vi "oa_TV Set Channel Info (Even Angle Output 1Chan).vi"(0 "seconds/rev":dbl[](array[numeric]) format="%.2f", 1 "torisional vibration unit (RPM)":enum16{"RPM", "deg/s", "rad/s"}(ring), 5 "pulse position":dbl[](array[numeric]), 7 "pulse/revolution (1)":i32=1, 11 "error in (no error)":errorcluster, 12 "r0":dbl, 13 "dr":dbl) -> (4 "even-angle torsional vibration":cluster{"r0":dbl, "dr":dbl, "Y":dbl[]}={"r0"=0.0, "dr"=1.0, "Y"=[]} {"r0" format="%.2p"; "dr" format="%.2p"; "Y" format="%.2f"}, 6 "even-angle channel info":T3={"channel name"="", "description"="", " channel info"={"sensor sensitivity"=1000.0, "engineering units"=1, "dB reference"=1.0, "custom label"="EU", "weighting filter"=0, "pregain"=0.0}} {"channel info"."pregain" format="%.2f"; "channel info"."weighting filter" items=["Linear", "A-weighting", "B-weighting", "C-weighting", "ITU-R 468-4", "Dolby", "CCITT", "C-message", "Wb", "Wc", "Wd", "We", "Wf", "Wh", "Wj", "Wk", "Wm", "AES17 20 kHz lowpass", "AES17 40 kHz lowpass", "AES17 20 kHz highpass", "AES17 40 kHz highpass"]; "channel info"."dB reference" format="%^.1e"; "channel info"."engineering units" items=["custom..."=0, "V"=1, "A"=21, "C"=30, "pC"=31, "s"=32, "-"=29, "Pa"=2, "N"=20, "g"=3, "m/s^2"=4, "m/s"=5, "m"=6, "mm/s"=12, "mm"=13, "micron/s"=14, "micron"=15, "in/s^2"=7, "in/s"=8, "in"=9, "mil/s"=10, "mil"=11, "rad/s^2"=16, "rad/s"=17, "rad"=18, "deg/s^2"=26, "deg/s"=27, "deg"=28, "RPM"=22, "cycle/s^2"=23, "Hz"=24, "cycle"=25, "strain"=19]; "channel info"."sensor sensitivity" format="%#_5f"}, 8 "speed profile":T2 {"speed [RPM]" format="%.2f"; "time [s]" format="%.2f"}, 10 "position info":T1, 14 "unit label":string, 15 "error out":errorcluster)   [LabVIEW 2017, in "SoundVib_Torsional.lvlib"]
uses:
  <vilib>/addons/Sound and Vibration/Order Analysis/Torsional Vibration/SoundVib_Torsional.lvlib
  <vilib>/addons/_NISVFA/_Shared subVIs/Controls/svc_Resampled Channel Info.ctl
  <vilib>/addons/_NISVFA/_Shared subVIs/Controls/svc_Channel Info.ctl
  <vilib>/addons/_NISVFA/_Shared subVIs/Controls/svc_Engineering Units Text Ring.ctl
  <vilib>/addons/_NISVFA/_Shared subVIs/Controls/svc_Weighting Filter Text Ring.ctl
  <vilib>/addons/Sound and Vibration/Order Analysis/Tach Process/SubVIs/speed profile.ctl
  <vilib>/addons/Sound and Vibration/Order Analysis/Misc/OAT Position Info.ctl
  <vilib>/addons/Sound and Vibration/Order Analysis/Tach Process/SoundVib_TachProcess.lvlib
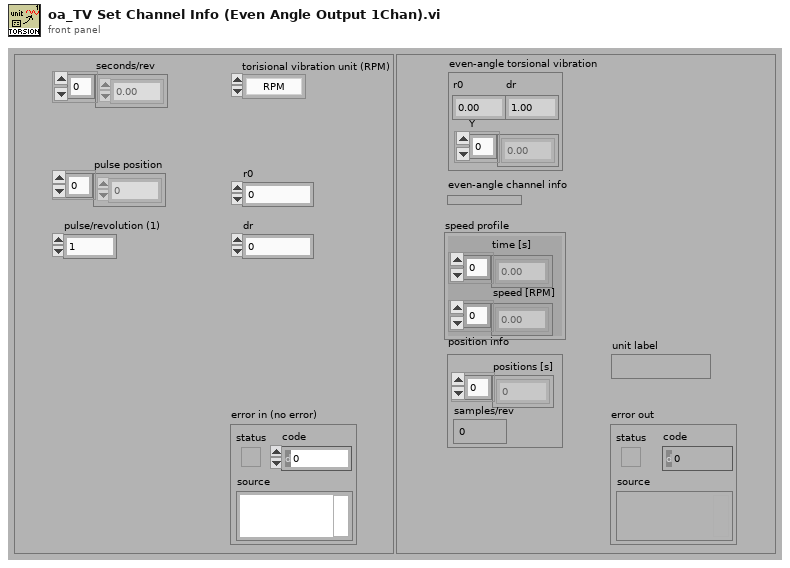
[diagram p1: front panel]
types:
  T1 = typedef "OAT Position Info.ctl" = cluster{"positions [s]":dbl[], "samples/rev":dbl}
  T2 = typedef "SoundVib_TachProcess.lvlib/speed profile.ctl" = cluster{"time [s]":dbl[], "speed [RPM]":dbl[]}
  T3 = typedef "svc_Resampled Channel Info.ctl" = cluster{"channel name":string, "description":string, " channel info":T4}
  T4 = typedef "svc_Channel Info.ctl" = cluster{"sensor sensitivity":dbl, "engineering units":T5, "dB reference":dbl, "custom label":string, "weighting filter":T6, "pregain":dbl}
  T5 = typedef "svc_Engineering Units Text Ring.ctl" = u16
  T6 = typedef "svc_Weighting Filter Text Ring.ctl" = u16
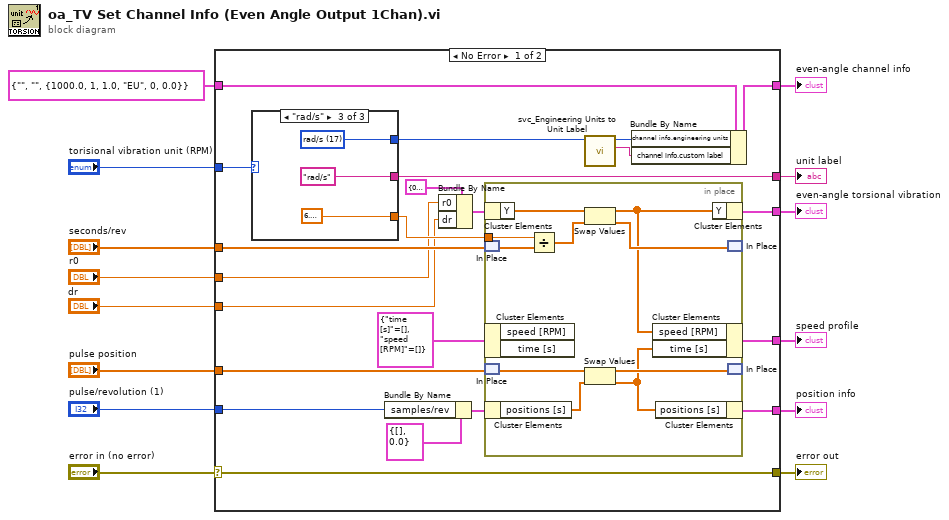
[diagram p0: block diagram]
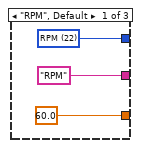
[diagram p2: hidden frame]
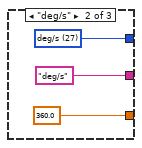
[diagram p3: hidden frame]
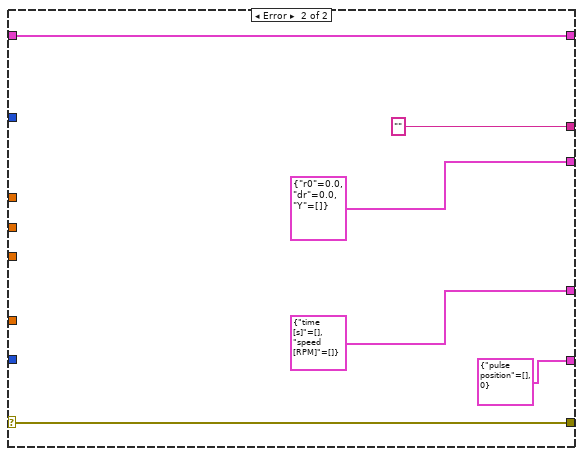
[diagram p4: hidden frame]
diagram:
  n1 = case shown="No Error" "error in (no error)" {
    selector: "error in (no error)" -> [w33 w59]
    tunnel: "torisional vibration unit (RPM)" -> [w35 _]
    tunnel: [w34 w55] -> w14
    tunnel: "seconds/rev" -> [w24 _]
    tunnel: "dr" -> [w20 _]
    tunnel: "r0" -> [w21 _]
    tunnel: [w31 cluster{"r0":dbl, "dr":dbl, "Y":dbl[]} {"r0"=0.0, "dr"=0.0, "Y"=[]} ("even-angle torsional vibration")] -> w10
    tunnel: [w33 w59] -> w8
    tunnel: [w32 ""] -> w6
    tunnel: "pulse position" -> [w27 _]
    tunnel: [w29 T2 {"time [s]"=[], "speed [RPM]"=[]} ("speed profile")] -> w4
    tunnel: "pulse/revolution (1)" -> [w16 _]
    tunnel: [w28 cluster{"pulse position":dbl[], i32} {"pulse position"=[], 0}] -> w2
    tunnel: T3 {"channel name"="", "description"="", " channel info"={"sensor sensitivity"=1000.0, "engineering units"=1, "dB reference"=1.0, "custom label"="EU", "weighting filter"=0, "pregain"=0.0}} ("even-angle channel info") -> [w22 w55]
    frame No Error {
      n2 = case shown="\"rad/s\"" w35 {
        tunnel: ["RPM" "deg/s" "rad/s"] -> w32
        tunnel: [60.0 ("even-time") 360.0 ("even-time") 6.283185307179586] -> w23
        tunnel: [w46 w49 w52] -> w26
        frame "RPM", Default {
          w46 = T5 22 items=["custom..."=0, "V"=1, "A"=21, "Pa"=2, "N"=20, "g"=3, "m/s^2"=4, "m/s"=5, "m"=6, "mm/s"=12, "mm"=13, "micron/s"=14, "micron"=15, "in/s^2"=7, "in/s"=8, "in"=9, "mil/s"=10, "mil"=11, "rad/s^2"=16, "rad/s"=17, "rad"=18, "deg/s^2"=26, "deg/s"=27, "deg"=28, "RPM"=22, "cycle/s^2"=23, "Hz"=24, "cycle"=25, "strain"=19] ("engineering units")
        }
        frame "deg/s" {
          w49 = T5 27 items=["custom..."=0, "V"=1, "A"=21, "Pa"=2, "N"=20, "g"=3, "m/s^2"=4, "m/s"=5, "m"=6, "mm/s"=12, "mm"=13, "micron/s"=14, "micron"=15, "in/s^2"=7, "in/s"=8, "in"=9, "mil/s"=10, "mil"=11, "rad/s^2"=16, "rad/s"=17, "rad"=18, "deg/s^2"=26, "deg/s"=27, "deg"=28, "RPM"=22, "cycle/s^2"=23, "Hz"=24, "cycle"=25, "strain"=19] ("engineering units")
        }
        frame "rad/s" {
          w52 = T5 17 items=["custom..."=0, "V"=1, "A"=21, "Pa"=2, "N"=20, "g"=3, "m/s^2"=4, "m/s"=5, "m"=6, "mm/s"=12, "mm"=13, "micron/s"=14, "micron"=15, "in/s^2"=7, "in/s"=8, "in"=9, "mil/s"=10, "mil"=11, "rad/s^2"=16, "rad/s"=17, "rad"=18, "deg/s^2"=26, "deg/s"=27, "deg"=28, "RPM"=22, "cycle/s^2"=23, "Hz"=24, "cycle"=25, "strain"=19] ("engineering units")
        }
      }
      n3 = Bundle By Name(cluster=T1 {"positions [s]"=[], "samples/rev"=0.0} ("position info"), "samples/rev"=w16) -> (w15:T1)
      n4 = Bundle By Name(cluster=cluster{"r0":dbl, "dr":dbl, "Y":dbl[]} {"r0"=0.0, "dr"=1.0, "Y"=[]} ("even-angle torsional vibration"), "r0"=w21, "dr"=w20) -> (w18:cluster{"r0":dbl, "dr":dbl, "Y":dbl[]})
      n5 = in-place {
        in-place-border: w23 -> [w44]
        n6 = in-place-cluster #1(w18) -> ("Y"=w43:dbl[])
        n7 = in-place-match #2(w24) -> (w45:dbl[])
        n8 = in-place-cluster #3(T2 {"time [s]"=[], "speed [RPM]"=[]} ("speed profile")) -> ()  [unwired: 2 out]
        n9 = in-place-match #4(w27) -> (w39:dbl[])
        n10 = in-place-cluster #5(w15) -> ("positions [s]"=w38:dbl[])
        n11 = Divide(x=w44, y=w45) -> (x/y=w42:dbl[])
        n12 = Swap Values(12:w43, 14:w42) -> (1:w40:dbl[], 3:w41:dbl[])  [unwired: 1 in]
        n13 = Swap Values(12:w39, 14:w38) -> (1:w37:dbl[], 3:w36:dbl[])  [unwired: 1 in]
        n14 = in-place-cluster #3("speed [RPM]"=w40, "time [s]"=w36) -> (w29:T2)
        n15 = in-place-cluster #5("positions [s]"=w36) -> (w28:T1)
        n16 = in-place-cluster #1("Y"=w40) -> (w31:cluster{"r0":dbl, "dr":dbl, "Y":dbl[]})
        n17 = in-place-match #2(w41) -> ()  [unwired: 1 out]
        n18 = in-place-match #4(w37) -> ()  [unwired: 1 out]
      }
      n19 = call <vilib>:"svc_Engineering Units to Unit Label.vi"("engineering units"=w26) -> ("unit label"=w25:string)  [unwired: 9 in, 1 out]
      n20 = Bundle By Name(cluster=w22, "channel info.engineering units"=w26, "channel info.custom label"=w25) -> (w34:T3)
    }
    frame Error {
    }
  }
  "even-angle channel info" <- w14
  "error out" <- w8
  "even-angle torsional vibration" <- w10
  "unit label" <- w6
  "speed profile" <- w4
  "position info" <- w2
